vi "xmlStringReadIng.vi"(4 "String":string) -> (1 "Value":i32)   [LabVIEW 2012]
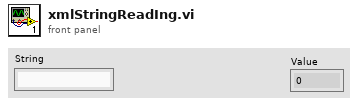
[diagram p1: front panel]
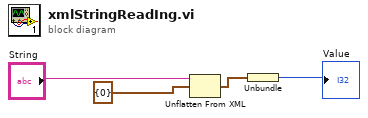
[diagram p0: block diagram]
diagram:
  n1 = Unflatten From XML(xml string="String", type=cluster{i32} {0}) -> (value=w3:cluster{i32})  [unwired: 1 in, 1 out]
  n2 = Unbundle(w3) -> (→"Value":i32)
